vi "ULx Read (Digital 1D Wfm NChan NSamp).vi"(0 "task in":refnum<k24>, 7 "number of samples per channel":i32=-1, 9 "timeout":dbl=10.0 format="%_4g", 11 "error in":errorcluster) -> (4 "task out":refnum<k24>, 6 "data":digitalwaveform[](array[waveform]), 15 "error out":errorcluster)   [LabVIEW 2020]
doc: "Reads one or more digital waveforms from a task that contains one or more digital input channels."
uses:
  C:/Users/William/Documents/LV 2020 builds/LeaktestDAQ/Source-v33/ULx_LV.dll
  ULx_LV.dll
panel:
  # "channel"
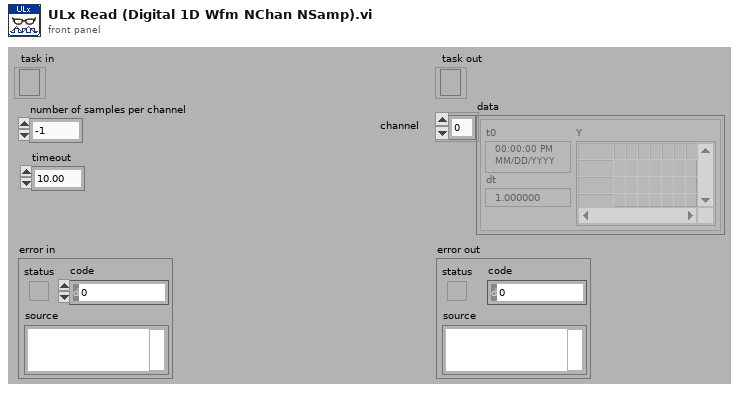
[diagram p1: front panel]
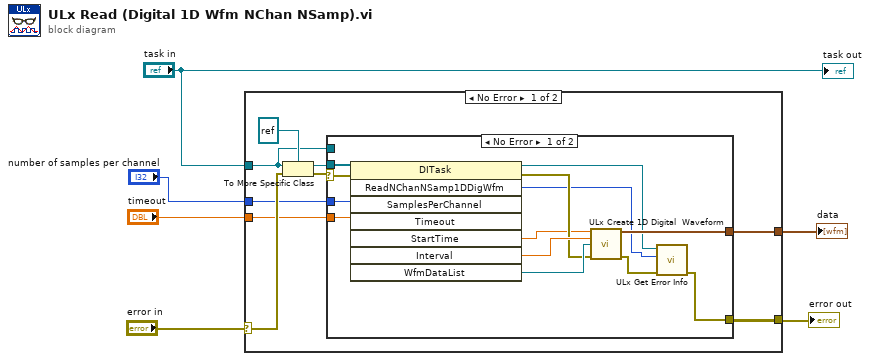
[diagram p0: block diagram]
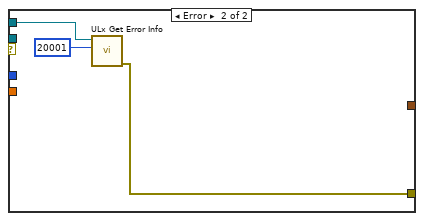
[diagram p2: hidden frame]
diagram:
  n1 = case shown="No Error" "error in" {
    selector: "error in" -> [w15 w32]
    tunnel: "task in" -> [w7 _]
    tunnel: "timeout" -> [w11 _]
    tunnel: [w10 w32] -> w4
    tunnel: "number of samples per channel" -> [w9 _]
    tunnel: [w8 _] -> w1
    frame No Error {
      n2 = To More Specific Class(target class=refnum<k24> refnum, reference=w7, error in=w15) -> (specific class reference=w12:refnum<k24>, error out=w13:errorcluster)
      n3 = case shown="No Error" w13 {
        selector: w13 -> [w27 _]
        tunnel: w12 -> [w28 _]
        tunnel: w11 -> [w26 _]
        tunnel: [w18 w29] -> w10
        tunnel: w9 -> [w25 _]
        tunnel: [w22 _] -> w8
        tunnel: w7 -> [_ w31]
        frame No Error {
          n4 = invoke class="DITask" method="ReadNChanNSamp1DDigWfm"(reference=w28, error in=w27, "SamplesPerChannel"=w25, "Timeout"=w26) -> (reference out=w21:refnum<k24>, error out=w20:errorcluster, "ReadNChanNSamp1DDigWfm"=w16:i32, "StartTime"=w17:dbl, "Interval"=w24:dbl, "WfmDataList"=w23:refnum<k24>)  [unwired: 4 in, 2 out]
          n5 = call "ULx Create 1D Digital  Waveform.vi"("t0"=w17, "dt"=w24, "data List"=w23, "error in"=w20) -> ("data"=w22:digitalwaveform[], "error out"=w19:errorcluster)  [unwired: 10 in]
          n6 = call "ULx Get Error Info.vi"("error in"=w19, "ErrorCode"=w16, "task in"=w21) -> ("error out"=w18:errorcluster)  [unwired: 8 in]
        }
        frame Error {
          n7 = call "ULx Get Error Info.vi"("ErrorCode"=20001, "task in"=w31) -> ("error out"=w29:errorcluster)  [unwired: 9 in]
        }
      }
    }
    frame Error {
    }
  }
  "error out" <- w4
  "data" <- w1
  "task out" <- "task in"
